vi "SQLite Delete Cycle Test.vi"(7 "Test DB Set Up Command":string, 8 "Error In (no error)":errorcluster, 11 "SQLite DB Operator In":refnum<class "SQLite DB Operator.lvclass">) -> (0 "Error Out":errorcluster, 3 "SQLite DB OperatorOut":refnum<class "SQLite DB Operator.lvclass">)   [LabVIEW 2023]
uses:
  Clasess/SQLite DB Operator/SQLite DB Operator.lvclass
  Clasess/DB Records/Expenses Tracker Cycle/Public/Ctrls/Cycle.ctl
  Clasess/DB Records/Expenses Tracker Cycle/Expenses Tracker Cycle.lvclass
  H:/Desktop/LabVIEW/LabView Repo/Expenses-Tracker-DB-Operator/Interfaces/Expenses Tracker Record/Expenses Tracker Record.lvclass
  Support/Editing/Edit Record Assert Error.vi
  Support/Editing/Edit Record Assert Not Error.vi
  <vilib>/drjdpowell/SQLite Library/SQL Connection/Execute SQL (1D Cluster).vi
  <vilib>/addons/_JKI Toolkits/Caraya/classes/Test/Test.lvclass
  <vilib>/drjdpowell/SQLite Library/SQLite.lvlib
  H:/Desktop/LabVIEW/LabView Repo/Expenses-Tracker-DB-Operator/Clasess/DB Records/Expenses Tracker Cycle/Expenses Tracker Cycle.lvclass
  <vilib>/drjdpowell/SQLite Library/SQL Connection/Connection.lvclass
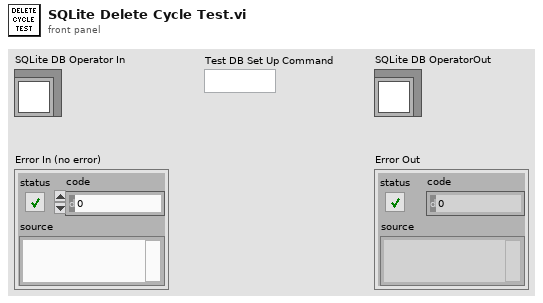
[diagram p1: front panel]
types:
  T1 = typedef "Expenses Tracker Cycle.lvclass/Cycle.ctl" = cluster{"ID":u32, "Name":string, "Day_of_occurence":u8, "Description":string}
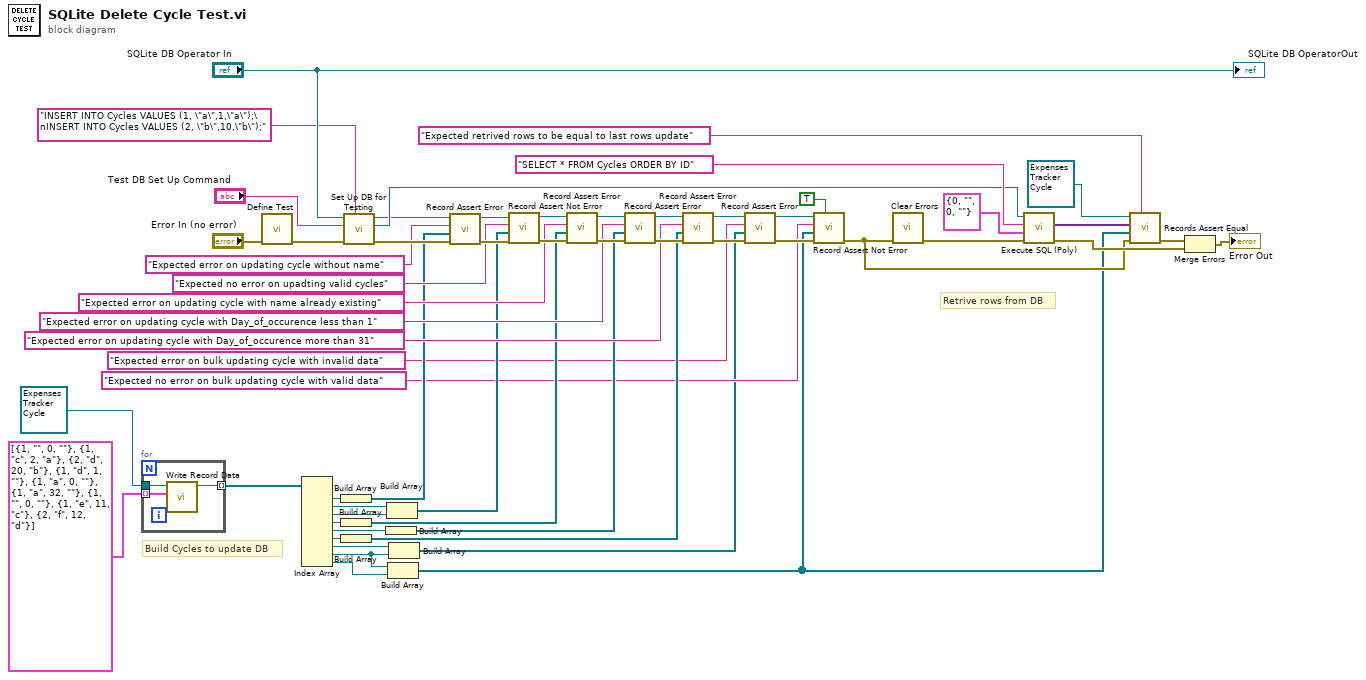
[diagram p0: block diagram]
diagram:
  # "Retrive rows from DB"
  # "Build Cycles to update DB"
  n1 = for {
    tunnel: T1[] [{"ID"=1, "Name"="", "Day_of_occurence"=0, "Description"=""}, {"ID"=1, "Name"="c", "Day_of_occurence"=2, "Description"="a"}, {"ID"=2, "Name"="d", "Day_of_occurence"=20, "Description"="b"}, {"ID"=1, "Name"="d", "Day_of_occurence"=1, "Description"=""}, {"ID"=1, "Name"="a", "Day_of_occurence"=0, "Description"=""}, {"ID"=1, "Name"="a", "Day_of_occurence"=32, "Description"=""}, {"ID"=1, "Name"="", "Day_of_occurence"=0, "Description"=""}, {"ID"=1, "Name"="e", "Day_of_occurence"=11, "Description"="c"}, {"ID"=2, "Name"="f", "Day_of_occurence"=12, "Description"="d"}] ("Array") -> [w60] mode=indexing
    tunnel: refnum<class "Expenses Tracker Cycle.lvclass"> refnum ("Expenses Tracker Category") -> [w59]
    tunnel: [w58] -> w54 mode=indexing
    n2 = call-dynamic "Write Record Data.vi"("Record"=w60, "Expenses Tracker Cycle In"=w59) -> ("Expenses Tracker Cycle Out"=w58:refnum<class "Expenses Tracker Cycle.lvclass">)  [unwired: 8 in, 1 out]
  }
  n3 = call <vilib>:"Define Test.vi"("error in (no error)"="Error In (no error)") -> ("error out"=w45:errorcluster)  [unwired: 9 in, 1 out]
  n4 = Index Array(array=w54) -> (element #1=w53:refnum<class "Expenses Tracker Cycle.lvclass">, element #2=w52:refnum<class "Expenses Tracker Cycle.lvclass">, element #3=w51:refnum<class "Expenses Tracker Cycle.lvclass">, element #4=w20:refnum<class "Expenses Tracker Cycle.lvclass">, element #5=w18:refnum<class "Expenses Tracker Cycle.lvclass">, element #6=w48:refnum<class "Expenses Tracker Cycle.lvclass">, element #7=w7:refnum<class "Expenses Tracker Cycle.lvclass">, element #8=w3:refnum<class "Expenses Tracker Cycle.lvclass">, element #9=w6:refnum<class "Expenses Tracker Cycle.lvclass">)  [unwired: 9 in]
  n5 = Build Array(w53) -> (w22:refnum<class "Expenses Tracker Cycle.lvclass">[])
  n6 = Build Array(w20) -> (w19:refnum<class "Expenses Tracker Cycle.lvclass">[])
  n7 = Build Array(w48) -> (w15:refnum<class "Expenses Tracker Cycle.lvclass">[])
  n8 = call "Set Up DB for Testing.vi"("Additional Set Up Commands"="INSERT INTO Cycles VALUES (1, \"a\",1,\"a\");\nINSERT INTO Cycles VALUES (2, \"b\",10,\"b\");", "Error In (no error)"=w45, "Test DB Set Up Command"="Test DB Set Up Command", "SQLite DB Operator In"="SQLite DB Operator In") -> ("Error Out"=w44:errorcluster, "SQLite Connection"=w47:refnum<class "Connection.lvclass">, "SQLite DB Operator Out"=w43:refnum<class "SQLite DB Operator.lvclass">)  [unwired: 5 in]
  n9 = Build Array(w18) -> (w17:refnum<class "Expenses Tracker Cycle.lvclass">[])
  n10 = Build Array(w52, w51) -> (w21:refnum<class "Expenses Tracker Cycle.lvclass">[])
  n11 = Build Array(w3, w6) -> (w4:refnum<class "Expenses Tracker Cycle.lvclass">[])
  n12 = Build Array(w7, w3) -> (w5:refnum<class "Expenses Tracker Cycle.lvclass">[])
  n13 = call-poly "Record Assert Error.vi"("Error In"=w44, "Records"=w22, "Assertion Label"="Expected error on updating cycle without name" ("Label (VI Title)"), "SQLite DB Operator In"=w43) -> ("Error Out"=w35:errorcluster, "SQLite DB Operator Out"=w34:refnum<class "SQLite DB Operator.lvclass">)  [unwired: 6 in]
  n14 = call-poly "Record Assert Not Error.vi"("Error In"=w35, "Records"=w21, "Assertion Label"="Expected no error on upadting valid cycles" ("Label (VI Title)"), "SQLite DB Operator In"=w34) -> ("Error Out"=w40:errorcluster, "SQLite DB Operator Out"=w41:refnum<class "SQLite DB Operator.lvclass">)  [unwired: 6 in]
  n15 = call-poly "Record Assert Error.vi"("Error In"=w40, "Records"=w19, "Assertion Label"="Expected error on updating cycle with name already existing" ("Label (VI Title)"), "SQLite DB Operator In"=w41) -> ("Error Out"=w38:errorcluster, "SQLite DB Operator Out"=w39:refnum<class "SQLite DB Operator.lvclass">)  [unwired: 6 in]
  n16 = call-poly "Record Assert Error.vi"("Error In"=w38, "Records"=w17, "Assertion Label"="Expected error on updating cycle with Day_of_occurence less than 1" ("Label (VI Title)"), "SQLite DB Operator In"=w39) -> ("Error Out"=w36:errorcluster, "SQLite DB Operator Out"=w37:refnum<class "SQLite DB Operator.lvclass">)  [unwired: 6 in]
  n17 = call-poly "Record Assert Error.vi"("Error In"=w36, "Records"=w15, "Assertion Label"="Expected error on updating cycle with Day_of_occurence more than 31" ("Label (VI Title)"), "SQLite DB Operator In"=w37) -> ("Error Out"=w14:errorcluster, "SQLite DB Operator Out"=w13:refnum<class "SQLite DB Operator.lvclass">)  [unwired: 6 in]
  n18 = call-poly "Record Assert Error.vi"("Error In"=w14, "Records"=w5, "Assertion Label"="Expected error on bulk updating cycle with invalid data" ("Label (VI Title)"), "SQLite DB Operator In"=w13) -> ("Error Out"=w11:errorcluster, "SQLite DB Operator Out"=w12:refnum<class "SQLite DB Operator.lvclass">)  [unwired: 6 in]
  n19 = call-poly "Record Assert Not Error.vi"("Bulk Update?"=TRUE, "Error In"=w11, "Records"=w4, "Assertion Label"="Expected no error on bulk updating cycle with valid data" ("Label (VI Title)"), "SQLite DB Operator In"=w12) -> ("Error Out"=w10:errorcluster)  [unwired: 5 in, 1 out]
  n20 = call <vilib>:"Clear Errors.vi"("error in (no error)"=w10) -> ("error out"=w25:errorcluster)  [unwired: 5 in, 1 out]
  n21 = call-poly <vilib>:"Execute SQL (Poly).vi"("error in (no error)"=w25, "Cluster (or Array of Clusters)"=T1 {"ID"=0, "Name"="", "Day_of_occurence"=0, "Description"=""} ("Cycle"), "SQL"="SELECT * FROM Cycles ORDER BY ID", "SQLite Connection in"=w47) -> ("error out"=w23:errorcluster, "Result Set (Array of Clusters)"=w28:variant[])  [unwired: 5 in, 1 out]
  n22 = call "Records Assert Equal.vi"("Assertion Label"="Expected retrived rows to be equal to last rows update" ("Label (VI Title)"), "Error In"=w10, "Correct Records"=w4, "Typedef Records"=w28, "Expenses Tracker Record In"=refnum<class "Expenses Tracker Cycle.lvclass"> refnum ("Expenses Tracker Category")) -> ("Error Out"=w24:errorcluster)  [unwired: 6 in]
  n23 = Merge Errors(w24, w23) -> (→"Error Out":errorcluster)
  "SQLite DB OperatorOut" <- "SQLite DB Operator In"
